vi "Move Impl.vi"(6 "Mode":enum16{"Relative", "Absolute"}(ring), 8 "error in (no error)":errorcluster, 9 "Value (um)":dbl format="%#_13g", 10 "Axis":T1=enum."Y", 11 "ASI Stage in":refnum<class "ASI Stage.lvclass">) -> (0 "error out":errorcluster, 3 "ASI Stage out":refnum<class "ASI Stage.lvclass">)   [LabVIEW 2023, in "ASI Stage.lvlib" / "ASI Stage.lvclass"]
uses:
  ASI Stage.lvclass
  Stage Controller/Stage Axis.ctl
  Stage Controller/Stage Controller.lvclass
  ASI Stage.lvclass/ASI Stage.ctl
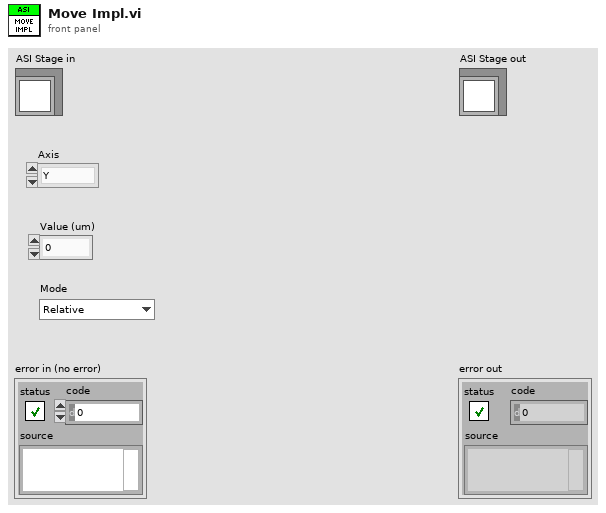
[diagram p1: front panel]
types:
  T1 = typedef "Stage Controller.lvlib/Stage Controller.lvclass/Stage Axis.ctl" = enum16{"unspecified", "X", "Y", "Z"}
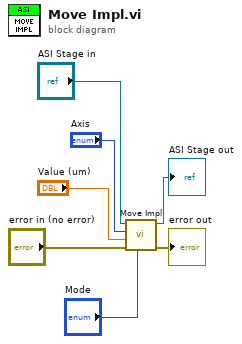
[diagram p0: block diagram]
diagram:
  n1 = call-parent "Move Impl.vi"("Mode"="Mode", "error in (no error)"="error in (no error)", "Value (um)"="Value (um)", "Axis"="Axis", "Stage Controller in"="ASI Stage in") -> ("error out"=→"error out":errorcluster, "Stage Controller out"=→"ASI Stage out":refnum<class "ASI Stage.lvclass">)  [unwired: 5 in]
